vi "Configure.vi"(8 "error in (no error)":errorcluster, 11 "navX - I2C in":refnum<class "navX - I2C.lvclass">) -> (0 "error out":errorcluster, 3 "navX - I2C out":refnum<class "navX - I2C.lvclass">)   [LabVIEW 2015, in "navX Library v3.lvlib" / "navX - I2C.lvclass"]
uses:
  navX - I2C.lvclass
  navX - I2C.lvclass/navX - I2C.ctl
  navX Registry Cache/_TypeDefs/DeviceRegistryTypeDef.ctl
  navX - Interface/_TypeDefs/CapabilityTypeDef.ctl
  navX - Interface/navX - Interface.lvclass/navX - Interface.ctl
  navX - Interface/navX - Interface.lvclass
  navX Registry Cache/navX Registry Cache.lvclass
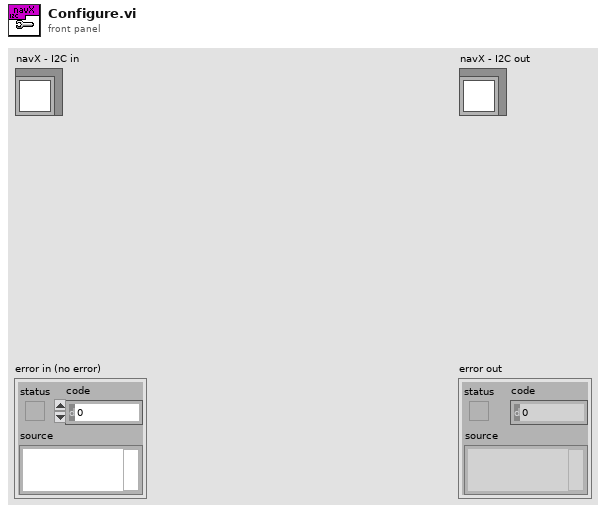
[diagram p1: front panel]
types:
  T1 = typedef "navX Library v3.lvlib/navX - Interface.lvclass/CapabilityTypeDef.ctl" = u16
  T2 = typedef "navX Library v3.lvlib/navX Registry Cache.lvclass/DeviceRegistryTypeDef.ctl" = u8
  T3 = typedef "WPI_I2CDevRef.ctl" = cluster{"DevStatus":errorcluster, "Device Address":u8, "Handle":i32, "I2C Bus":T4}
  T4 = typedef "i2c_bus.ctl" = enum16{"I2C On-Board", "I2C MXP", "Invalid"}
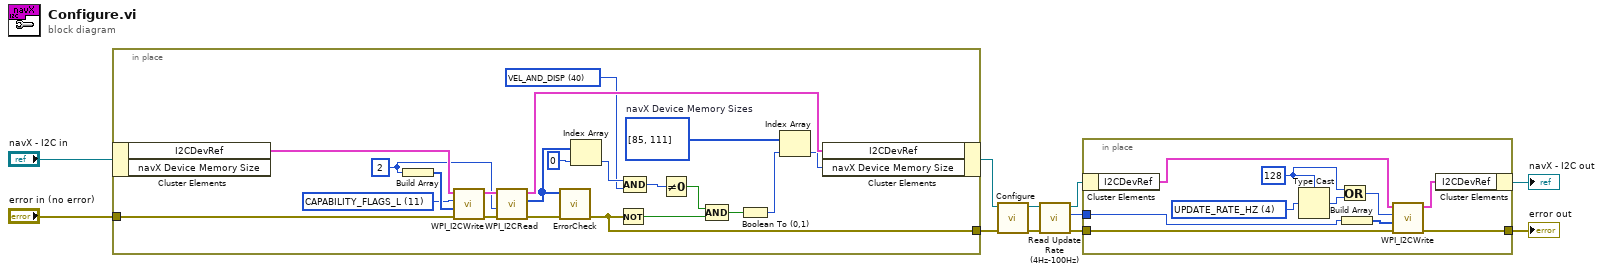
[diagram p0: block diagram]
diagram:
  n1 = in-place {
    in-place-border: [w13] -> w6
    in-place-border: "error in (no error)" -> [w29]
    w21 = i32[] [85, 111]  # navX Device Memory Sizes
    w24 = T1 40 items=["OMNIMOUNT"=4, "OMNIMOUNT_CONFIG_MASK"=38, "VEL_AND_DISP"=40, "YAW_RESET"=80] ("Capability Flag")
    w19 = u8 2 ("hex")
    w20 = T2 11 items=["WHOAMI"=0, "HW_REV"=1, "FW_VER_MAJOR"=2, "FW_VER_MINOR"=3, "UPDATE_RATE_HZ"=4, "ACCEL_FSR_G"=5, "GYRO_FSR_DPS"=6, "OP_STATUS"=8, "CAL_STATUS"=9, "SELFTEST_STATUS"=10, "CAPABILITY_FLAGS_L"=11, "CAPABILITY_FLAGS_H"=12, "SENSOR_STATUS"=16, "TIMESTAMP"=18, "YAW"=22, "ROLL"=24, "PITCH"=26, "HEADING"=28, "FUSED_HEADING"=30, "ALTITUDE_I"=32, "ALTITUDE_D"=34, "LINERA_ACC_X"=36, "LINERA_ACC_Y"=38, "LINERA_ACC_Z"=40, "QUAT_W"=42, "QUAT_X"=44, "QUAT_Y"=46, "QUAT_Z"=48, "MPU_TEMP_C"=50, "GYRO_X"=52, "GYRO_Y"=54, "GYRO_Z"=56, "ACC_X"=58, "ACC_Y"=60, "ACC_Z"=62, "MAG_X"=64, "MAG_Y"=66, "MAG_Z"=68, "PRESSURE_I"=70, "PRESSURE_D"=72, "PRESSURE_TEMP"=74, "YAW_OFFSET"=76, "QUAT_OFFSET_W"=78, "QUAT_OFFSET_X"=80, "QUAT_OFFSET_Y"=82, "QUAT_OFFSET_Z"=84, "INTEGRATION_CONTROL"=86, "VELOCITY_X"=88, "VELOCITY_Y"=92, "VELOCITY_Z"=96, "DISPLACMENT_X"=100, "DISPLACMENT_Y"=104, "DISPLACEMENT_Z"=108] ("Device Register")
    n2 = in-place-cluster #1("navX - I2C in") -> ("I2CDevRef"=w30:T3)  [unwired: 1 out]
    n3 = Build Array(w19) -> (w27:u8[])
    n4 = call <vilib>:"WPI_I2CWrite.vi"("error in (no error)"=w29, "I2CDataToSend"=w27, "I2CRegister"=w20, "I2CDevRef"=w30) -> ("error out"=w32:errorcluster, "I2CDevRef"=w31:T3)  [unwired: 6 in]
    n5 = call <vilib>:"WPI_I2CRead.vi"("error in (no error)"=w32, "I2CBytesToRead"=w19, "I2CDevRef"=w31) -> ("error out"=w15:errorcluster, "Data Out"=w16:u8[], "I2CDevRef"=w28:T3)  [unwired: 6 in]
    n6 = call "ErrorCheck.vi"("error in (no error)"=w15, "I2C Data in"=w16) -> ("error out"=w13:errorcluster)  [unwired: 9 in]
    n7 = Index Array(array=w16, index=0) -> (element=w25:u8)
    n8 = Not(x=w13) -> (.not. x?=w12:bool)
    n9 = Compound Arithmetic op=AND(w25, w24) -> (w23:T1)
    n10 = Not Equal To 0?(x=w23) -> (x != 0?=w18:bool)
    n11 = Compound Arithmetic op=AND(w18, w12) -> (w14:bool)
    n12 = Boolean To (0,1)(Boolean=w14) -> (0, 1=w22:i16)
    n13 = Index Array(array=w21, index=w22) -> (element=w17:i32)
    n14 = in-place-cluster #1("I2CDevRef"=w28, "navX Device Memory Size"=w17) -> (w3:refnum<class "navX - I2C.lvclass">)
  }
  n15 = call-parent "Configure.vi"("error in (no error)"=w6, "navX - Base in"=w3) -> ("error out"=w5:errorcluster, "navX - Base out"=w4:refnum<class "navX - I2C.lvclass">)  [unwired: 8 in]
  n16 = call "Read Update Rate (4Hz-100Hz).vi"("error in (no error)"=w5, "navX - Base in"=w4) -> ("error out"=w9:errorcluster, "Update Rate (4Hz-100Hz)"=w10:u8, "navX - Base out"=w2:refnum<class "navX - I2C.lvclass">)  [unwired: 7 in]
  n17 = in-place {
    in-place-border: [w37] -> w11
    in-place-border: w10 -> [w36]
    in-place-border: w9 -> [w35]
    w41 = u8 128
    w40 = T2 4 items=["WHOAMI"=0, "HW_REV"=1, "FW_VER_MAJOR"=2, "FW_VER_MINOR"=3, "UPDATE_RATE_HZ"=4, "ACCEL_FSR_G"=5, "GYRO_FSR_DPS"=6, "OP_STATUS"=8, "CAL_STATUS"=9, "SELFTEST_STATUS"=10, "CAPABILITY_FLAGS_L"=11, "CAPABILITY_FLAGS_H"=12, "SENSOR_STATUS"=16, "TIMESTAMP"=18, "YAW"=22, "ROLL"=24, "PITCH"=26, "HEADING"=28, "FUSED_HEADING"=30, "ALTITUDE_I"=32, "ALTITUDE_D"=34, "LINERA_ACC_X"=36, "LINERA_ACC_Y"=38, "LINERA_ACC_Z"=40, "QUAT_W"=42, "QUAT_X"=44, "QUAT_Y"=46, "QUAT_Z"=48, "MPU_TEMP_C"=50, "GYRO_X"=52, "GYRO_Y"=54, "GYRO_Z"=56, "ACC_X"=58, "ACC_Y"=60, "ACC_Z"=62, "MAG_X"=64, "MAG_Y"=66, "MAG_Z"=68, "PRESSURE_I"=70, "PRESSURE_D"=72, "PRESSURE_TEMP"=74, "YAW_OFFSET"=76, "QUAT_OFFSET_W"=78, "QUAT_OFFSET_X"=80, "QUAT_OFFSET_Y"=82, "QUAT_OFFSET_Z"=84, "INTEGRATION_CONTROL"=86, "VELOCITY_X"=88, "VELOCITY_Y"=92, "VELOCITY_Z"=96, "DISPLACMENT_X"=100, "DISPLACMENT_Y"=104, "DISPLACEMENT_Z"=108] ("Device Register")
    n18 = in-place-cluster #2(w2) -> ("I2CDevRef"=w34:T3)
    n19 = Type Cast(type=w41, x=w40) -> (*(type *) &x=w42:u8)
    n20 = Or(x=w41, y=w42) -> (x .or. y?=w38:u8)
    n21 = Build Array(w36) -> (w39:u8[])
    n22 = call <vilib>:"WPI_I2CWrite.vi"("error in (no error)"=w35, "I2CDataToSend"=w39, "I2CRegister"=w38, "I2CDevRef"=w34) -> ("error out"=w37:errorcluster, "I2CDevRef"=w33:T3)  [unwired: 6 in]
    n23 = in-place-cluster #2("I2CDevRef"=w33) -> (→"navX - I2C out":refnum<class "navX - I2C.lvclass">)
  }
  "error out" <- w11
